vi "C37 Scale Phasor Signals.vi"(7 "Phasor Scaling":T1, 10 "Phasor Value Imaginary (or angle)":sgl[](array[numeric]), 11 "Phasor Value Real (or amplitude)":sgl[](array[numeric])) -> (3 "Phasor Values":csg[](array[numeric]), 5 "Polar Flag":bool)   [LabVIEW 2018, in "S3DK.lvlib" / "C37118-DLL.lvlib"]
uses:
  C37118-DLL.lvlib
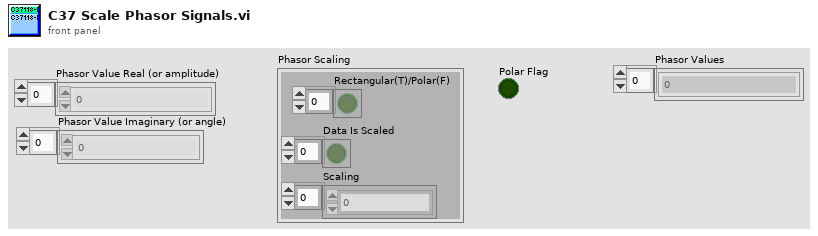
[diagram p1: front panel]
types:
  T1 = cluster{"Rectangular(T)/Polar(F)":bool[], "Data Is Scaled":bool[], "Scaling":sgl[]}
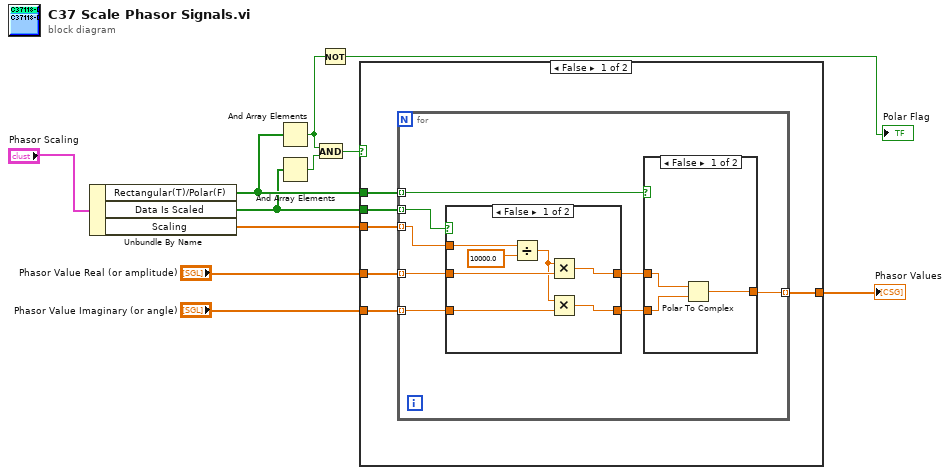
[diagram p0: block diagram]
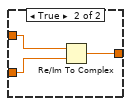
[diagram p2: hidden frame]
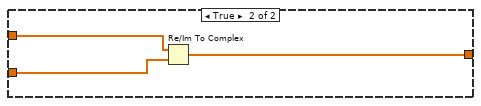
[diagram p4: hidden frame]
diagram:
  n1 = Unbundle By Name("Phasor Scaling") -> ("Rectangular(T)/Polar(F)"=w7:bool[], "Data Is Scaled"=w6:bool[], "Scaling"=w9:sgl[])
  n2 = And Array Elements(Boolean array=w7) -> (logical AND=w5:bool)
  n3 = And Array Elements(Boolean array=w6) -> (logical AND=w4:bool)
  n4 = And(x=w5, y=w4) -> (x .and. y?=w3:bool)
  n5 = Not(x=w5) -> (.not. x?=→"Polar Flag":bool)
  n6 = case shown="False" w3 {
    tunnel: "Phasor Value Real (or amplitude)" -> [w17 w43]
    tunnel: "Phasor Value Imaginary (or angle)" -> [w16 w42]
    tunnel: w9 -> [w15 _]
    tunnel: w7 -> [w14 _]
    tunnel: w6 -> [w13 _]
    tunnel: [w12 w41] -> w2
    frame False {
      n7 = for {
        tunnel: w17 -> [w25] mode=indexing
        tunnel: w16 -> [w24] mode=indexing
        tunnel: w15 -> [w21] mode=indexing
        tunnel: w13 -> [w22] mode=indexing
        tunnel: w14 -> [w18] mode=indexing
        tunnel: [w23] -> w12 mode=indexing
        n8 = case shown="False" w22 {
          tunnel: w25 -> [w36 w40]
          tunnel: w24 -> [w35 w39]
          tunnel: w21 -> [w38 _]
          tunnel: [w33 w39] -> w20
          tunnel: [w32 w40] -> w19
          frame False {
            n9 = Divide(x=w38, y=sgl 10000.0) -> (x/y=w34:sgl)
            n10 = Multiply(x=w34, y=w36) -> (x*y=w32:sgl)
            n11 = Multiply(x=w34, y=w35) -> (x*y=w33:sgl)
          }
          frame True {
          }
        }
        n12 = case shown="False" w18 {
          tunnel: [w26 w31] -> w23
          tunnel: w20 -> [w27 w29]
          tunnel: w19 -> [w28 w30]
          frame False {
            n13 = Polar To Complex(1:w27, 2:w28) -> (0:w26:csg)
          }
          frame True {
            n14 = Re/Im To Complex(1:w29, 2:w30) -> (0:w31:csg)
          }
        }
      }
    }
    frame True {
      n15 = Re/Im To Complex(1:w42, 2:w43) -> (0:w41:csg[])
    }
  }
  "Phasor Values" <- w2
